vi "Read Buffer Count.vi"(8 "error in":errorcluster, 11 "VISA resource name":refnum<visa-resource-name>) -> (0 "error out":errorcluster, 1 "Confirmation Response":string, 3 "VISA resource name out":refnum<visa-resource-name>)   [LabVIEW 2024, in "Micron Optics sm130.lvlib"]
uses:
  Micron Optics sm130.lvlib
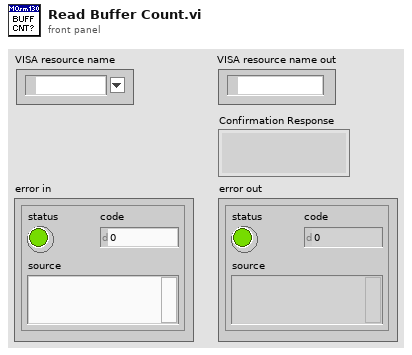
[diagram p1: front panel]
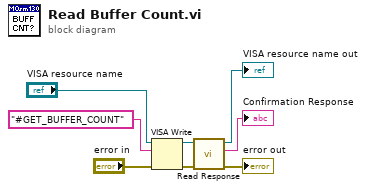
[diagram p0: block diagram]
diagram:
  n1 = VISA Write(VISA resource name="VISA resource name", write buffer="#GET_BUFFER_COUNT" ("string"), error in (no error)="error in") -> (VISA resource name out=w5:refnum<visa-resource-name>, error out=w4:errorcluster)  [unwired: 1 out]
  n2 = call "Read Response.vi"("error in (no error)"=w4, "VISA resource name"=w5) -> ("error out"=→"error out":errorcluster, "Confirmation Response"=→"Confirmation Response":string, "VISA resource name out"=→"VISA resource name out":refnum<visa-resource-name>)  [unwired: 7 in]
